vi "Remove Sr No header.vi"(11 "Column Headers[] in":string[](array[string])) -> (3 "Column Headers[] out":string[](array[string]))   [LabVIEW 2018]
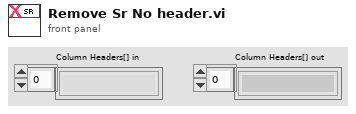
[diagram p1: front panel]
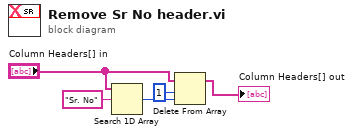
[diagram p0: block diagram]
diagram:
  n1 = Search 1D Array(1D array="Column Headers[] in", element="Sr. No") -> (index of element=w2:i32)  [unwired: 1 in]
  n2 = Delete From Array(array="Column Headers[] in", length=1, index=w2) -> (array with subset deleted=→"Column Headers[] out":string[])  [unwired: 1 out]
